vi "imp_test_v2.vi"() -> ()   [LabVIEW 2014]
uses:
  <vilib>/LabVIEW Targets/FPGA/cRIO/shared/nicrio_ModuleControls/nicrio_cRIO-9237_DataRatesRing.ctl
  <vilib>/LabVIEW Targets/FPGA/cRIO/shared/nicrio_ModuleControls/nicrio_cRIO-9237_ExcitationVoltageRing.ctl
  <vilib>/rvi/FXPMathLib/FxpSinAndCos/subVIs/nifxpmath_SinAndCos_SimConfig.ctl
  <vilib>/rvi/Emulation/niFpgaGetClockAttributes.vi
  <vilib>/rvi/Emulation/niFpgaSctlEmulationGetInTimedLoop.vi
  <vilib>/rvi/Emulation/niFpgaEmulationReportErrorSimple.vi
  <vilib>/rvi/Emulation/niFpgaProcessEmulError.vi
  <vilib>/rvi/interface/RandomDataEmulation/nirviRandomDataMultiElementFPGAFIFO.vi
  <instcachedir>/0/nirviRandomDataMultiElementFPGAFIFO_AD0CFC12EF974623A9C2E4184BC062B2.lvgen/nirviRandomDataMultiElementFPGAFIFO_AD0CFC12EF974623A9C2E4184BC062B2_023.vi
  <vilib>/rvi/interface/RandomDataEmulation/niFpgaRandomDataHandleErrors.vi
  <vilib>/rvi/Emulation/niFpgaCriticalErrorInLSC.vi
  <vilib>/rvi/eio/common/nirviEmuTemplateMethod_errors.vi
  <vilib>/rvi/FXPMathLib/FxpSinAndCos/simVIs/DllFxpSinAndCosTemp_sub.vi
  <vilib>/rvi/eio/common/nirviEmuTemplatePropertySet_errors.vi
  <vilib>/rvi/DataTransferAndStorage/Container/XNode/niFpgaContainer.xnode
  <vilib>/rvi/interface/RandomDataEmulation/nirviRandomDataFpgaMultiElementTemplate.vi
  <vilib>/eio/EIONode/EIONode.xnode
  <vilib>/rvi/FXPMathLib/FxpMul/XNode/nifxpmath_Multiplier.xnode
  <vilib>/rvi/FXPMathLib/FxpSinAndCos/XNode/nifxpmath_SinAndCos.xnode
  <vilib>/rvi/Analysis/measure/butterworth/XNode/niFpgaButterworthFilter.xnode
  <vilib>/rvi/FXPMathLib/FxpSub/XNode/nifxpmath_Sub.xnode
  <vilib>/rvi/FXPMathLib/FxpAdd/XNode/nifxpmath_Add.xnode
  <vilib>/eio/EIOPropertyNode/EIOPropertyNode.xnode
  <vilib>/rvi/eio/common/nirviEmuTemplatePropertyGet_errors.vi
  <vilib>/rvi/eio/common/nirviEmuTemplatePropertyGet_noerrors.vi
  <vilib>/rvi/eio/common/nirviEmuTemplatePropertySet_noerrors.vi
  <vilib>/rvi/FXPMathLib/sim/FxpSim.dll
panel:
  out "Strain (mean)":fxp<+/-,32,4>
  in  "Strain selection":i16(ring) items=["Raw strain", "Mean strain", "Filtered strain"]
  in  "ft_d or dt_d2":i16(ring) items=["ft_d", "ft_d2"]
  out "vb":fxp<+/-,38,8>
  out "va":fxp<+/-,38,8>
  out "ft_d2":fxp<+/-,64,59>
  out "Force_r":fxp<+/-,64,42>
  in  "Bv":fxp<+/-,22,8>
  out "D_error_dd":fxp<+/-,64,49>
  out "D_error_d":fxp<+/-,33,10>
  in  "Kv":fxp<+/-,22,8>
  out "D_error":fxp<+/-,64,33>
  out "Dr_sin_dd":fxp<+/-,64,48>
  out "Dr_sin_d":fxp<+/-,64,17>
  out "Sin omega":fxp<+/-,52,9>
  out "Dr_sin":fxp<+/-,39,10>
  in  "Sin offset":fxp<+/-,38,9>
  in  "Sin magnitude":fxp<+/-,22,7>
  out "Time now(s)":fxp<+,52,14>
  in  "Sin wave freq. (Hz)":fxp<+/-,32,6>
  in  "Dr":fxp<+/-,22,7>
  in  "Drive mode":i16(ring) items=["Backward", "Forward"]
  in  "ft_d coeff.":i32[](array[numeric])=[946630756, 63555534]
  out "ft_d":fxp<+/-,36,25>
  out "D_dd":fxp<+/-,36,24>
  in  "D_dd coeff.":i32[](array[numeric])=[946630756, 63555534]
  out "dF_PID":fxp<+/-,36,33>
  in  "dF_PID coeff.":i32[](array[numeric])=[946630756, 63555534]
  out "ft_i":fxp<+/-,34,18>
  out "F_PID":fxp<+/-,51,14>
  in  "f_tolorance":fxp<+,22,6>
  in  "Ki":fxp<+/-,36,9>
  in  "Kd":fxp<+/-,36,9>
  out "f_tilde":fxp<+/-,33,11>
  in  "Kp":fxp<+/-,36,9>
  out "vq_F":fxp<+/-,20,5> format="%.57g"
  out "vd_F":fxp<+/-,20,5>
  in  "dF_add":bool
  out "D_d(mm/s)":fxp<+/-,41,10>
  out "omega(rad/s)":fxp<+/-,20,9>
  in  "Veolcity Estimation":i16(ring) items=["T method", "M_avg method", "M method"]
  in  "Stop motor":bool
  out "D_d(T)":fxp<+/-,41,10>
  out "omega(T)":fxp<+/-,20,9>
  in  "mt0_omega":u32
  out "mt_omega":u32
  out "rad(NrTheta)":fxp<+/-,33,10>
  out "D(mm)":fxp<+/-,32,10>
  out "Encoder Position":i32
  in  "Encoder reset":bool
  in  "Ini coe.":bool
  out "Loop rate (kHz)":fxp<+/-,36,7>
  in  "Strain filter coeff.":i32[](array[numeric])=[-850883994, 1909449570, 3794062, -975456236, 2033039520, 4039635]
  out "Force":fxp<+/-,32,10>
  out "Strain (filter)":fxp<+/-,36,4>
  out "Fileterd data":fxp<+/-,32,4>
  in  "S/F coeff":fxp<+/-,20,-12>
  out "Raw Strain":fxp<+/-,36,4>
  in  "Strain gage reset":bool
  in  "Stop (Strain)":bool
  out "Mod6/AI2":fxp<+/-,32,4>
  in  "Shunt Cal Enable":bool
  in  "Half-Bridge Enable":bool
  in  "Excitation Voltage":T1 items=["2.5 Volts", "3.3 Volts", "5.0 Volts", "10.0 Volts", "External Excitation"]
  in  "Data Rate":T2=1 items=["50.000 kS/s (NI 9237)"=1, "25.000 kS/s (NI 9237)"=2, "16.667 kS/s (NI 9237)"=3, "12.500 kS/s (NI 9237)"=4, "10.000 kS/s (NI 9237)"=5, "8.333 kS/s (NI 9237)"=6, "7.143 kS/s (NI 9237)"=7, "6.250 kS/s (NI 9237)"=8, "5.556 kS/s (NI 9237)"=9, "5.000 kS/s (NI 9237)"=10, "4.545 kS/s (NI 9237)"=11, "4.167 kS/s (NI 9237)"=12, "3.846 kS/s (NI 9237)"=13, "3.571 kS/s (NI 9237)"=14, "3.333 kS/s (NI 9237)"=15, "3.125 kS/s (NI 9237)"=16, "2.941 kS/s (NI 9237)"=17, "2.778 kS/s (NI 9237)"=18, "2.632 kS/s (NI 9237)"=19, "2.500 kS/s (NI 9237)"=20, "2.381 kS/s (NI 9237)"=21, "2.273 kS/s (NI 9237)"=22, "2.174 kS/s (NI 9237)"=23, "2.083 kS/s (NI 9237)"=24, "2.000 kS/s (NI 9237)"=25, "1.923 kS/s (NI 9237)"=26, "1.852 kS/s (NI 9237)"=27, "1.786 kS/s (NI 9237)"=28, "1.724 kS/s (NI 9237)"=29, "1.667 kS/s (NI 9237)"=30, "1.613 kS/s (NI 9237)"=31]
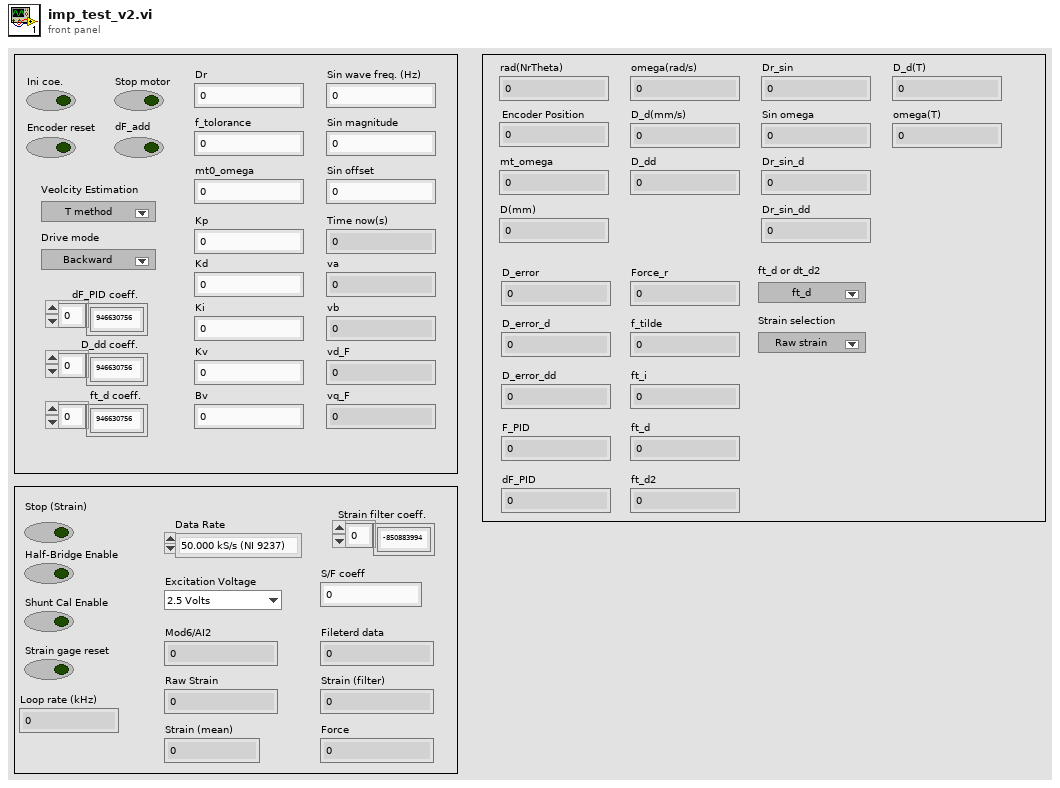
[diagram p1: front panel]
types:
  T1 = typedef "nicrio_cRIO-9237_ExcitationVoltageRing.ctl" = u8
  T2 = typedef "nicrio_cRIO-9237_DataRatesRing.ctl" = u8
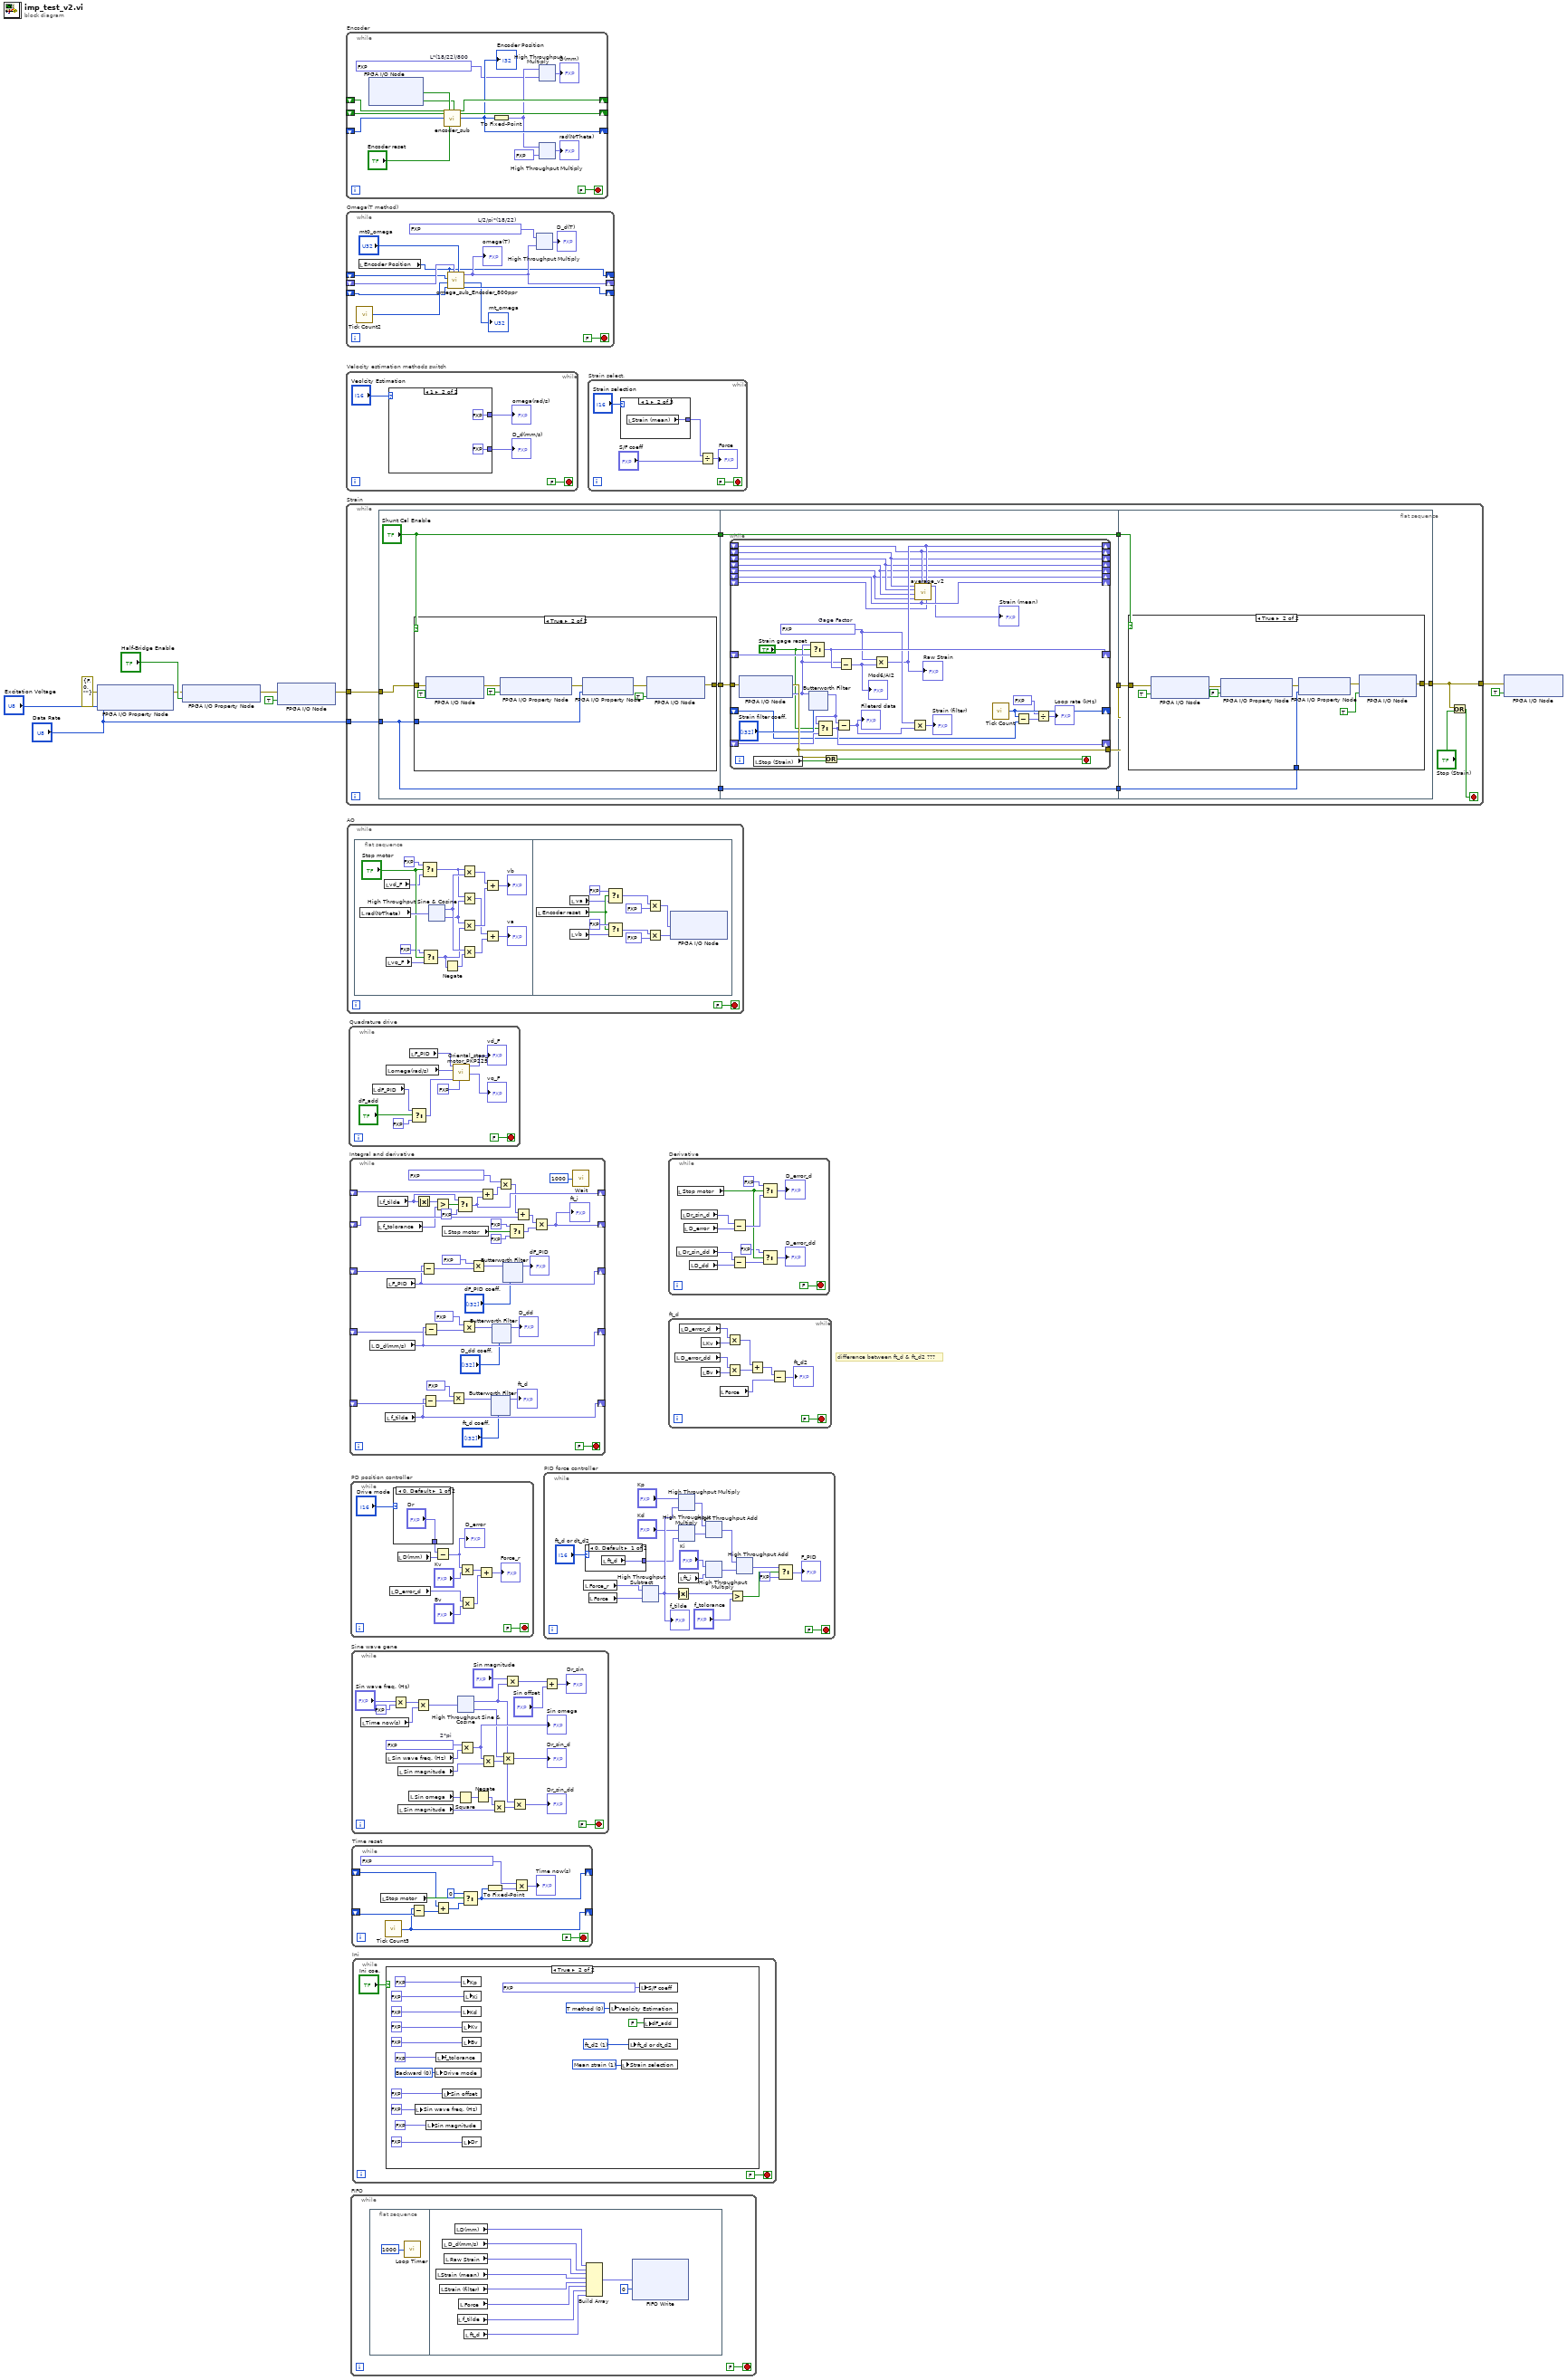
[diagram p0: block diagram]
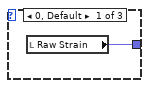
[diagram p2: hidden frame]
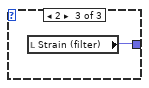
[diagram p3: hidden frame]
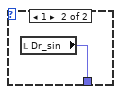
[diagram p4: hidden frame]
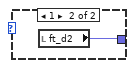
[diagram p5: hidden frame]
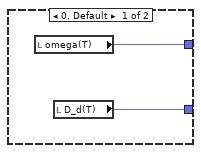
[diagram p6: hidden frame]
diagram:
  # "difference between ft_d & ft_d2 ???"
  n1 = xnode "FPGA I/O Property Node"("error in"=errorcluster {"status"=FALSE, "code"=0, "source"=""}, "Data Rate"="Data Rate", "Excitation Voltage"="Excitation Voltage") -> ("error out"=w7:errorcluster)  [unwired: 1 in, 1 out]
  n2 = xnode "FPGA I/O Property Node"("error in"=w7, "Half-Bridge Enable"="Half-Bridge Enable") -> ("error out"=w6:errorcluster)  [unwired: 1 in, 1 out]
  n3 = xnode "FPGA I/O Node"("error in"=w6, "Mod6/Start"=TRUE) -> ("error out"=w4:errorcluster)  [unwired: 1 in, 1 out]
  n4 = while "Encoder" {
    shift-right: [w22] -> _
    shift-left: _ -> [w23]
    shift-right: [w24] -> _
    shift-left: _ -> [w25]
    shift-right: [w17] -> _
    shift-left: _ -> [w21]
    stop <- FALSE stop-if-true
    w14 = fxp<+/-,32,0> 0.0020454544574022293  # L*(18/22)/800
    n5 = xnode "FPGA I/O Node"() -> ("Mod4/DI3"=w20:bool, "Mod4/DI4"=w19:bool)  [unwired: 2 in, 2 out]
    n6 = call "encoder_sub.vi"("A_pre"=w23, "B_pre"=w25, "Encoder Position_pre"=w21, "A input"=w20, "Encoder Position Reset"="Encoder reset", "B input"=w19) -> ("A"=w22:bool, "B"=w24:bool, "Encoder Position (Counts)"=w17:i32)  [unwired: 19 in]
    "Encoder Position" <- w17
    n7 = To Fixed-Point(number=w17) -> (fixed-point=w16:fxp<+/-,32,32>)  [unwired: 1 in]
    n8 = xnode ("High Throughput Multiply")("x"=w16, "y"=w14) -> ("x*y"=→"D(mm)":fxp<+/-,64,32>)
    n9 = xnode ("High Throughput Multiply")("x"=w16, "y"=fxp<+/-,16,1> 0.125) -> ("x*y"=→"rad(NrTheta)":fxp<+/-,48,33>)
  }
  n10 = while "Omega(T method)" {
    shift-right: [w27] -> _
    shift-left: _ -> [w28]
    shift-right: [w31] -> _
    shift-left: _ -> [w33]
    shift-right: [w35] -> _
    shift-left: _ -> [w36]
    stop <- FALSE stop-if-true
    w30 = fxp<+/-,32,0> 0.2604353614151478  # L/2/pi*(18/22)
    n11 = call "Tick Count2"() -> ("Tick Count(Ticks)"=w37:u32)
    n12 = local read "Encoder Position"() -> (w27:i32)
    n13 = call "omega_sub_Encoder_800ppr.vi"("mt0"="mt0_omega", "omega_pre"=w33, "ticks_m_pre"=w36, "ticks"=w37, "count_pre"=w28, "count"=w27) -> ("ticks_m"=w35:u32, "mt"=→"mt_omega":u32, "omega"=w31:fxp<+/-,20,9>)  [unwired: 3 in]
    "omega(T)" <- w31
    n14 = xnode ("High Throughput Multiply")("x"=w30, "y"=w31) -> ("x*y"=→"D_d(T)":fxp<+/-,52,9>)
  }
  n15 = while "Velocity estimation methods switch" {
    stop <- FALSE stop-if-true
    n16 = case shown="1" "Veolcity Estimation" {
      tunnel: [w43 fxp<+/-,20,9> 0.0 ("omega(T)")] -> w40
      tunnel: [w42 fxp<+/-,41,10> 0.0 ("D_d(T)")] -> w39
      frame 0, Default {
        n17 = local read "omega(T)"() -> (w43:fxp<+/-,20,9>)
        n18 = local read "D_d(T)"() -> (w42:fxp<+/-,41,10>)
      }
      frame 1 {
      }
    }
    "omega(rad/s)" <- w40
    "D_d(mm/s)" <- w39
  }
  n19 = while "Strain" {
    tunnel: w4 -> [w56]
    tunnel: "Data Rate" -> [w55]
    tunnel: [w47] -> w2
    stop <- w48 stop-if-true
    n20 = flat-sequence {
      tunnel: w56 -> [w60]
      tunnel: w55 -> [w59]
      tunnel: [w59] -> w54
      tunnel: ["Shunt Cal Enable"] -> w53
      tunnel: [w57] -> w52
      tunnel: w54 -> [w72]
      tunnel: w53 -> [w73]
      tunnel: w52 -> [w74]
      tunnel: [w73] -> w51
      tunnel: [w71] -> w50
      tunnel: [w72] -> w49
      tunnel: w51 -> [w116]
      tunnel: w50 -> [w115]
      tunnel: w49 -> [w114]
      tunnel: [w113] -> w47
      frame #0 {
        n21 = case shown="True" "Shunt Cal Enable" {
          tunnel: w60 -> [w61 w68]
          tunnel: w59 -> [_ w66]
          tunnel: [w61 w63] -> w57
          frame False {
          }
          frame True {
            n22 = xnode "FPGA I/O Node"("error in"=w68, "Mod6/Stop"=TRUE) -> ("error out"=w69:errorcluster)  [unwired: 1 in, 1 out]
            n23 = xnode "FPGA I/O Property Node"("error in"=w69, "Shunt Cal Enable"=TRUE) -> ("error out"=w67:errorcluster)  [unwired: 1 in, 1 out]
            n24 = xnode "FPGA I/O Property Node"("error in"=w67, "Data Rate"=w66) -> ("error out"=w65:errorcluster)  [unwired: 1 in, 1 out]
            n25 = xnode "FPGA I/O Node"("error in"=w65, "Mod6/Start"=TRUE) -> ("error out"=w63:errorcluster)  [unwired: 1 in, 1 out]
          }
        }
      }
      frame #1 {
        n26 = while {
          tunnel: w74 -> [w104]
          tunnel: [w102] -> w71
          shift-right: [w100] -> _
          shift-left: _ -> [w101]
          shift-right: [w96] -> _
          shift-left: _ -> [w97]
          shift-right: [w88] -> _
          shift-left: _ -> [w89]
          shift-right: [w83] -> _
          shift-left: _ -> [w82]
          shift-right: [w82] -> _
          shift-left: _ -> [w81]
          shift-right: [w81] -> _
          shift-left: _ -> [w80]
          shift-right: [w80] -> _
          shift-left: _ -> [w79]
          shift-right: [w79] -> _
          shift-left: _ -> [w78]
          shift-right: [w78] -> _
          shift-left: _ -> [w77]
          shift-right: [w77] -> _
          shift-left: _ -> [w76]
          stop <- w91 stop-if-true
          w94 = fxp<+,20,2> 2.115001678466797  # Gage Factor
          n27 = xnode "FPGA I/O Node"("error in"=w104) -> ("error out"=w102:errorcluster, "Mod6/AI2"=w98:fxp<+/-,24,-4>)  [unwired: 1 in, 1 out]
          n28 = local read "Stop (Strain)"() -> (w103:bool)
          n29 = xnode "Butterworth Filter"("input data"=w98, "scaled coefficients"="Strain filter coeff.") -> ("output data"=w95:fxp<+/-,28,0>)  [unwired: 1 in]
          n30 = Select(t=w98, s="Strain gage reset", f=w101) -> (s? t:f=w100:fxp<+/-,24,-4>)
          n31 = Select(t=w95, s="Strain gage reset", f=w97) -> (s? t:f=w96:fxp<+/-,28,0>)
          n32 = Or(x=w102, y=w103) -> (x .or. y?=w91:bool)
          n33 = Subtract(x=w95, y=w96) -> (x-y=w93:fxp<+/-,32,16>)
          "Fileterd data" <- w93
          n34 = Subtract(x=w98, y=w100) -> (x-y=w99:fxp<+/-,25,-3>)
          "Mod6/AI2" <- w99
          n35 = Multiply(x=w94, y=w99) -> (x*y=w83:fxp<+/-,41,6>)
          "Raw Strain" <- w83
          n36 = Multiply(x=w94, y=w93) -> (x*y=→"Strain (filter)":fxp<+/-,41,6>)
          n37 = call "average_v2.vi"("Numeric 8"=w76, "Numeric"=w83, "Numeric 7"=w77, "Numeric 2"=w82, "Numeric 6"=w78, "Numeric 5"=w79, "Numeric 4"=w80, "Numeric 3"=w81) -> ("mean"=→"Strain (mean)":fxp<+/-,32,4>)  [unwired: 2 in, 1 out]
          n38 = call "Tick Count"() -> ("Tick Count(uSec)"=w88:u32)
          n39 = Subtract(x=w88, y=w89) -> (x-y=w86:fxp<+/-,32,16>)
          n40 = Divide(x=fxp<+,7,10> 1000.0, y=w86) -> (x/y=→"Loop rate (kHz)":fxp<+/-,40,27>)
        }
      }
      frame #2 {
        n41 = case shown="True" w116 {
          tunnel: w115 -> [w117 w125]
          tunnel: w114 -> [_ w121]
          tunnel: [w117 w118] -> w113
          frame False {
          }
          frame True {
            n42 = xnode "FPGA I/O Node"("error in"=w125, "Mod6/Stop"=TRUE) -> ("error out"=w123:errorcluster)  [unwired: 1 in, 1 out]
            n43 = xnode "FPGA I/O Property Node"("error in"=w123, "Shunt Cal Enable"=FALSE) -> ("error out"=w122:errorcluster)  [unwired: 1 in, 1 out]
            n44 = xnode "FPGA I/O Property Node"("error in"=w122, "Data Rate"=w121) -> ("error out"=w120:errorcluster)  [unwired: 1 in, 1 out]
            n45 = xnode "FPGA I/O Node"("error in"=w120, "Mod6/Start"=TRUE) -> ("error out"=w118:errorcluster)  [unwired: 1 in, 1 out]
          }
        }
      }
    }
    n46 = Or(x=w47, y="Stop (Strain)") -> (x .or. y?=w48:bool)
  }
  n47 = while "AO" {
    stop <- FALSE stop-if-true
    n48 = flat-sequence {
      frame #0 {
        n49 = local read "rad(NrTheta)"() -> (w144:fxp<+/-,33,10>)
        n50 = local read "vd_F"() -> (w142:fxp<+/-,20,5>)
        n51 = local read "vq_F"() -> (w141:fxp<+/-,20,5>)
        n52 = Select(t=fxp<+/-,20,5> 0.0, s="Stop motor", f=w142) -> (s? t:f=w136:fxp<+/-,20,5>)
        n53 = Select(t=fxp<+/-,20,5> 0.0, s="Stop motor", f=w141) -> (s? t:f=w135:fxp<+/-,20,5>)
        n54 = xnode "High Throughput Sine & Cosine"("x (pi)"=w144) -> ("sin(x)"=w138:fxp<+/-,17,2>, "cos(x)"=w137:fxp<+/-,17,2>)
        n55 = Negate(x=w135) -> (-x=w134:fxp<+/-,21,6>)
        n56 = Multiply(x=w136, y=w138) -> (x*y=w133:fxp<+/-,37,7>)
        n57 = Multiply(x=w136, y=w137) -> (x*y=w131:fxp<+/-,37,7>)
        n58 = Multiply(x=w137, y=w135) -> (x*y=w132:fxp<+/-,37,7>)
        n59 = Multiply(x=w138, y=w134) -> (x*y=w130:fxp<+/-,36,6>)
        n60 = Add(x=w133, y=w132) -> (x+y=→"vb":fxp<+/-,38,8>)
        n61 = Add(x=w131, y=w130) -> (x+y=→"va":fxp<+/-,37,7>)
      }
      frame #1 {
        n62 = local read "Encoder reset"() -> (w177:bool)
        n63 = local read "vb"() -> (w175:fxp<+/-,38,8>)
        n64 = local read "va"() -> (w176:fxp<+/-,38,8>)
        n65 = Select(t=fxp<+,2,2> 3.0, s=w177, f=w176) -> (s? t:f=w181:fxp<+/-,38,8>)
        n66 = Select(t=fxp<+,1,1> 0.0, s=w177, f=w175) -> (s? t:f=w180:fxp<+/-,38,8>)
        n67 = Multiply(x=w181, y=fxp<+/-,1,0> -0.5) -> (x*y=w184:fxp<+/-,39,8>)
        n68 = Multiply(x=w180, y=fxp<+/-,1,0> -0.5) -> (x*y=w185:fxp<+/-,37,6>)
        n69 = xnode "FPGA I/O Node"("Mod8/AO2"=w184, "Mod8/AO3"=w185) -> ()  [unwired: 2 in, 2 out]
      }
    }
  }
  n70 = while "Quadrature drive" {
    stop <- FALSE stop-if-true
    n71 = local read "dF_PID"() -> (w187:fxp<+/-,36,33>)
    n72 = local read "omega(rad/s)"() -> (w195:fxp<+/-,20,9>)
    n73 = local read "F_PID"() -> (w188:fxp<+/-,51,14>)
    n74 = Select(t=w187, s="dF_add", f=fxp<+,1,1> 0.0) -> (s? t:f=w191:fxp<+/-,36,33>)
    n75 = call "Oriental_step_motor_PKP225.vi"("F_Threshold"=fxp<+,12,12> 10.0, "dFmr"=w191, "omega"=w195, "Fmr"=w188) -> ("vq_F"=→"vq_F":fxp<+/-,20,5>, "vd_F"=→"vd_F":fxp<+/-,20,5>)  [unwired: 6 in]
  }
  n76 = while "Integral and derivative" {
    shift-right: [w227] -> _
    shift-left: _ -> [w226]
    shift-right: [w219] -> _
    shift-left: _ -> [w218]
    shift-right: [w229] -> _
    shift-left: _ -> [w230]
    shift-right: [w209] -> _
    shift-left: _ -> [w208]
    shift-right: [w201] -> _
    shift-left: _ -> [w205]
    stop <- FALSE stop-if-true
    n77 = local read "D_d(mm/s)"() -> (w209:fxp<+/-,41,10>)
    n78 = local read "f_tolorance"() -> (w197:fxp<+,22,6>)
    n79 = local read "f_tilde"() -> (w231:fxp<+/-,33,11>)
    n80 = local read "f_tilde"() -> (w201:fxp<+/-,33,11>)
    n81 = local read "F_PID"() -> (w229:fxp<+/-,51,14>)
    n82 = Absolute Value(x=w231) -> (abs(x)=w233:fxp<+,33,11>)
    n83 = Subtract(x=w229, y=w230) -> (x-y=w217:fxp<+/-,52,15>)
    n84 = Subtract(x=w201, y=w205) -> (x-y=w204:fxp<+/-,34,12>)
    n85 = Subtract(x=w209, y=w208) -> (x-y=w211:fxp<+/-,42,11>)
    n86 = Greater?(x=w233, y=w197) -> (0:w234:bool)
    n87 = local read "Stop motor"() -> (w220:bool)
    n88 = Multiply(x=fxp<+/-,33,11> 1000.0, y=w204) -> (x*y=w202:fxp<+/-,64,22>)
    n89 = Select(t=w231, s=w234, f=fxp<+/-,33,11> 0.0) -> (s? t:f=w227:fxp<+/-,33,11>)
    n90 = Multiply(x=fxp<+,7,10> 1000.0, y=w211) -> (x*y=w210:fxp<+/-,49,21>)
    n91 = Multiply(x=fxp<+/-,52,15> 1000.0, y=w217) -> (x*y=w214:fxp<+/-,64,29>)
    n92 = Add(x=w226, y=w227) -> (x+y=w232:fxp<+/-,34,12>)
    n93 = xnode "Butterworth Filter"("input data"=w202, "scaled coefficients"="ft_d coeff.") -> ("output data"=→"ft_d":fxp<+/-,36,26>)  [unwired: 1 in]
    n94 = xnode "Butterworth Filter"("input data"=w210, "scaled coefficients"="D_dd coeff.") -> ("output data"=→"D_dd":fxp<+/-,36,25>)  [unwired: 1 in]
    n95 = Multiply(x=fxp<+/-,30,12> 0.000499725341796875, y=w232) -> (x*y=w225:fxp<+/-,64,24>)
    n96 = xnode "Butterworth Filter"("input data"=w214, "scaled coefficients"="dF_PID coeff.") -> ("output data"=→"dF_PID":fxp<+/-,36,33>)  [unwired: 1 in]
    n97 = Select(t=fxp<+,1,1> 0.0, s=w220, f=fxp<+,1,1> 1.0) -> (s? t:f=w223:fxp<+,1,1>)
    n98 = Add(x=w225, y=w218) -> (x+y=w224:fxp<+/-,64,24>)
    n99 = Multiply(x=w224, y=w223) -> (x*y=w219:fxp<+/-,34,18>)
    "ft_i" <- w219
    n100 = call "Wait"("Count(uSec)"=u32 1000) -> ()  [unwired: 1 out]
  }
  n101 = while "PD position controller" {
    stop <- FALSE stop-if-true
    n102 = local read "D_error_d"() -> (w263:fxp<+/-,33,10>)
    n103 = case shown="0, Default" "Drive mode" {
      tunnel: ["Dr" w272] -> w268
      frame 0, Default {
      }
      frame 1 {
        n104 = local read "Dr_sin"() -> (w272:fxp<+/-,39,10>)
      }
    }
    n105 = local read "D(mm)"() -> (w269:fxp<+/-,32,10>)
    n106 = Subtract(x=w268, y=w269) -> (x-y=w267:fxp<+/-,40,11>)
    "D_error" <- w267
    n107 = Multiply(x=w267, y="Kv") -> (x*y=w265:fxp<+/-,61,18>)
    n108 = Multiply(x=w263, y="Bv") -> (x*y=w262:fxp<+/-,55,18>)
    n109 = Add(x=w265, y=w262) -> (x+y=→"Force_r":fxp<+/-,62,19>)
  }
  n110 = while "FIFO" {
    stop <- FALSE stop-if-true
    n111 = flat-sequence {
      frame #0 {
        n112 = call "Loop Timer"("Count(uSec)"=u32 1000) -> ()  [unwired: 1 out]
      }
      frame #1 {
        n113 = local read "Strain (mean)"() -> (w281:fxp<+/-,32,4>)
        n114 = local read "Strain (filter)"() -> (w280:fxp<+/-,36,4>)
        n115 = local read "D_d(mm/s)"() -> (w283:fxp<+/-,41,10>)
        n116 = local read "Raw Strain"() -> (w282:fxp<+/-,36,4>)
        n117 = local read "D(mm)"() -> (w284:fxp<+/-,32,10>)
        n118 = local read "f_tilde"() -> (w278:fxp<+/-,33,11>)
        n119 = local read "Force"() -> (w279:fxp<+/-,32,10>)
        n120 = local read "ft_d"() -> (w275:fxp<+/-,36,25>)
        n121 = Build Array(w284, w283, w282, w281, w280, w279, w278, w275) -> (w277:fxp<+/-,57,25>[])
        n122 = xnode ("FIFO Write")("Element"=w277, "Timeout"=0) -> ()  [unwired: 1 in, 2 out]
      }
    }
  }
  n123 = while "Sine wave gene" {
    stop <- FALSE stop-if-true
    w299 = fxp<+,20,3> 6.2831878662109375  # 2*pi
    n124 = local read "Time now(s)"() -> (w305:fxp<+,52,14>)
    n125 = local read "Sin wave freq. (Hz)"() -> (w298:fxp<+/-,32,6>)
    n126 = Multiply(x="Sin wave freq. (Hz)", y=fxp<+/-,32,6> 2.0) -> (x*y=w306:fxp<+/-,64,12>)
    n127 = local read "Sin magnitude"() -> (w296:fxp<+/-,22,7>)
    n128 = local read "Sin magnitude"() -> (w289:fxp<+/-,22,7>)
    n129 = local read "Sin omega"() -> (w292:fxp<+/-,52,9>)
    n130 = Multiply(x=w306, y=w305) -> (x*y=w304:fxp<+/-,64,25>)
    n131 = Square(x=w292) -> (x^2=w291:fxp<+,64,16>)
    n132 = xnode "High Throughput Sine & Cosine"("x (pi)"=w304) -> ("sin(x)"=w286:fxp<+/-,16,2>, "cos(x)"=w294:fxp<+/-,16,2>)
    n133 = Multiply(x=w299, y=w298) -> (x*y=w297:fxp<+/-,52,9>)
    "Sin omega" <- w297
    n134 = Negate(x=w291) -> (-x=w290:fxp<+/-,64,17>)
    n135 = Multiply(x=w297, y=w296) -> (x*y=w295:fxp<+/-,64,15>)
    n136 = Multiply(x=w290, y=w289) -> (x*y=w288:fxp<+/-,64,24>)
    n137 = Multiply(x=w294, y=w295) -> (x*y=→"Dr_sin_d":fxp<+/-,64,17>)
    n138 = Multiply(x="Sin magnitude", y=w286) -> (x*y=w302:fxp<+/-,38,9>)
    n139 = Multiply(x=w286, y=w288) -> (x*y=→"Dr_sin_dd":fxp<+/-,64,26>)
    n140 = Add(x=w302, y="Sin offset") -> (x+y=→"Dr_sin":fxp<+/-,39,10>)
  }
  n141 = while "Time reset" {
    shift-right: [w348] -> _
    shift-left: _ -> [w349]
    shift-right: [w343] -> _
    shift-left: _ -> [w344]
    stop <- FALSE stop-if-true
    n142 = local read "Stop motor"() -> (w350:bool)
    n143 = call "Tick Count3"() -> ("Tick Count(uSec)"=w348:u32)
    n144 = Subtract(x=w348, y=w349) -> (x-y=w347:u32)
    n145 = Add(x=w344, y=w347) -> (x+y=w346:u32)
    n146 = Select(t=u32 0, s=w350, f=w346) -> (s? t:f=w343:u32)
    n147 = To Fixed-Point(number=w343) -> (fixed-point=w342:fxp<+,32,32>)  [unwired: 1 in]
    n148 = Multiply(x=fxp<+,20,-18> 1.0000003385357559e-06, y=w342) -> (x*y=→"Time now(s)":fxp<+,52,14>)
  }
  n149 = while "Ini" {
    stop <- FALSE stop-if-true
    n150 = case shown="True" "Ini coe." {
      frame False {
      }
      frame True {
        w353 = i16 1 items=["Raw strain", "Mean strain", "Filtered strain"] ("Strain selection")
        w354 = i16 1 items=["ft_d", "ft_d2"] ("ft_d or dt_d2")
        w360 = i16 0 items=["T method", "M_avg method", "M method"] ("Veolcity Estimation")
        w362 = i16 0 items=["Backward", "Forward"] ("Drive mode")
        n151 = local write "Sin wave freq. (Hz)"(fxp<+/-,32,6> 1.0 ("Sin wave freq. (Hz)")) -> ()
        n152 = local write "Sin magnitude"(fxp<+/-,22,7> 10.0 ("Sin magnitude")) -> ()
        n153 = local write "Drive mode"(w362) -> ()
        n154 = local write "f_tolorance"(fxp<+,22,6> 10.0 ("f_tolorance")) -> ()
        n155 = local write "Sin offset"(fxp<+/-,38,9> 0.0 ("Sin offset")) -> ()
        n156 = local write "Kp"(fxp<+/-,36,9> 50.0 ("Kp")) -> ()
        n157 = local write "Kd"(fxp<+/-,36,9> 0.0 ("Kd")) -> ()
        n158 = local write "Kv"(fxp<+/-,22,8> 1.0 ("Kv")) -> ()
        n159 = local write "Bv"(fxp<+/-,22,8> 0.0 ("Bv")) -> ()
        n160 = local write "Dr"(fxp<+/-,22,7> 0.0 ("Dr")) -> ()
        n161 = local write "Ki"(fxp<+/-,36,9> 0.0 ("Ki")) -> ()
        n162 = local write "Veolcity Estimation"(w360) -> ()
        n163 = local write "Strain selection"(w353) -> ()
        n164 = local write "ft_d or dt_d2"(w354) -> ()
        n165 = local write "S/F coeff"(fxp<+/-,41,4> 1.047803380060941e-06 ("S/F coeff")) -> ()
        n166 = local write "dF_add"(FALSE ("dF_add")) -> ()
      }
    }
  }
  n167 = while "PID force controller" {
    stop <- FALSE stop-if-true
    n168 = local read "Force_r"() -> (w373:fxp<+/-,64,42>)
    n169 = case shown="0, Default" "ft_d or dt_d2" {
      tunnel: [w389 w390] -> w369
      frame 0, Default {
        n170 = local read "ft_d"() -> (w389:fxp<+/-,36,25>)
      }
      frame 1 {
        n171 = local read "ft_d2"() -> (w390:fxp<+/-,64,59>)
      }
    }
    n172 = local read "Force"() -> (w387:fxp<+/-,32,10>)
    n173 = xnode "High Throughput Subtract"("x"=w373, "y"=w387) -> ("x-y"=w386:fxp<+/-,64,43>)
    "f_tilde" <- w386
    n174 = Absolute Value(x=w386) -> (abs(x)=w377:fxp<+,64,43>)
    n175 = local read "ft_i"() -> (w372:fxp<+/-,34,18>)
    n176 = xnode ("High Throughput Multiply")("x"="Kp", "y"=w386) -> ("x*y"=w384:fxp<+/-,64,52>)
    n177 = xnode ("High Throughput Multiply")("x"="Kd", "y"=w369) -> ("x*y"=w383:fxp<+/-,64,68>)
    n178 = xnode ("High Throughput Add")("x"=w384, "y"=w383) -> ("x+y"=w380:fxp<+/-,64,69>)
    n179 = xnode ("High Throughput Multiply")("x"="Ki", "y"=w372) -> ("x*y"=w381:fxp<+/-,64,27>)
    n180 = Greater?(x=w377, y="f_tolorance") -> (0:w375:bool)
    n181 = xnode ("High Throughput Add")("x"=w380, "y"=w381) -> ("x+y"=w379:fxp<+/-,64,70>)
    n182 = Select(t=w379, s=w375, f=fxp<+/-,51,14> 0.0) -> (s? t:f=→"F_PID":fxp<+/-,64,70>)
  }
  n183 = while "Strain select." {
    stop <- FALSE stop-if-true
    n184 = case shown="1" "Strain selection" {
      tunnel: [w396 w397 w398] -> w393
      frame 0, Default {
        n185 = local read "Raw Strain"() -> (w396:fxp<+/-,36,4>)
      }
      frame 1 {
        n186 = local read "Strain (mean)"() -> (w397:fxp<+/-,32,4>)
      }
      frame 2 {
        n187 = local read "Strain (filter)"() -> (w398:fxp<+/-,36,4>)
      }
    }
    n188 = Divide(x=w393, y="S/F coeff") -> (x/y=→"Force":fxp<+/-,32,10>)
  }
  n189 = while "Derivative" {
    stop <- FALSE stop-if-true
    n190 = local read "Dr_sin_dd"() -> (w404:fxp<+/-,64,48>)
    n191 = local read "Stop motor"() -> (w402:bool)
    n192 = local read "Dr_sin_d"() -> (w407:fxp<+/-,64,17>)
    n193 = local read "D_error"() -> (w408:fxp<+/-,64,33>)
    n194 = local read "D_dd"() -> (w405:fxp<+/-,36,24>)
    n195 = Subtract(x=w407, y=w408) -> (x-y=w406:fxp<+/-,64,34>)
    n196 = Subtract(x=w404, y=w405) -> (x-y=w403:fxp<+/-,64,49>)
    n197 = Select(t=fxp<+,1,1> 0.0, s=w402, f=w406) -> (s? t:f=→"D_error_d":fxp<+/-,64,34>)
    n198 = Select(t=fxp<+/-,64,49> 0.0, s=w402, f=w403) -> (s? t:f=→"D_error_dd":fxp<+/-,64,49>)
  }
  n199 = while "ft_d" {
    stop <- FALSE stop-if-true
    n200 = local read "D_error_dd"() -> (w417:fxp<+/-,64,49>)
    n201 = local read "D_error_d"() -> (w419:fxp<+/-,33,10>)
    n202 = local read "Kv"() -> (w420:fxp<+/-,22,8>)
    n203 = local read "Bv"() -> (w418:fxp<+/-,22,8>)
    n204 = local read "Force"() -> (w413:fxp<+/-,32,10>)
    n205 = Multiply(x=w419, y=w420) -> (x*y=w415:fxp<+/-,55,18>)
    n206 = Multiply(x=w417, y=w418) -> (x*y=w416:fxp<+/-,64,57>)
    n207 = Add(x=w415, y=w416) -> (x+y=w414:fxp<+/-,64,58>)
    n208 = Subtract(x=w414, y=w413) -> (x-y=→"ft_d2":fxp<+/-,64,59>)
  }
  n209 = xnode "FPGA I/O Node"("error in"=w2, "Mod6/Stop"=TRUE) -> ()  [unwired: 1 in, 2 out]
